vi "CRC-16.vi"(6 "Reflected":bool, 8 "FinalXorValue":u16 format="%04x", 9 "InitialCRC":u16 format="%04x", 10 "Polynomial":u16 format="%04x", 11 "DATA":u8[](array[numeric]) format="%02x") -> (3 "CRC":u16 format="%04x")   [LabVIEW 2021, in "LIN Frame Protection Addon Engine.lvlib"]
uses:
  LIN Frame Protection Addon Engine.lvlib
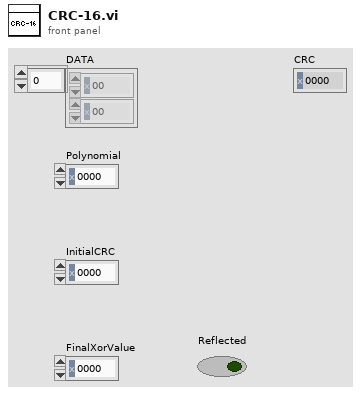
[diagram p1: front panel]
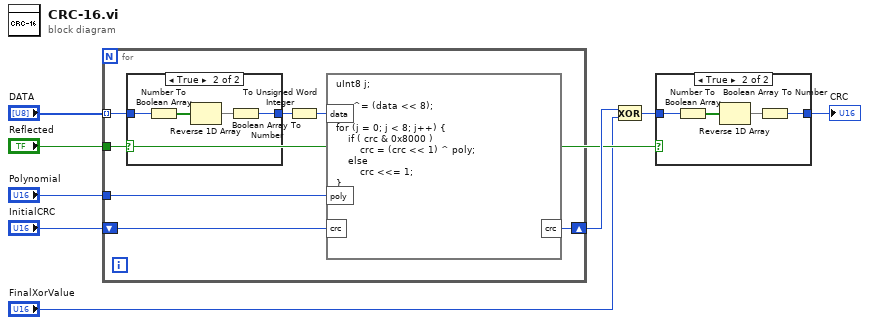
[diagram p0: block diagram]
diagram:
  n1 = for {
    tunnel: "Polynomial" -> [w15]
    tunnel: "DATA" -> [w11] mode=indexing
    tunnel: "Reflected" -> [w13]
    shift-right: [w10] -> w5
    shift-left: "InitialCRC" -> [w14]
    n2 = case shown="True" w13 {
      tunnel: [w16 w19] -> w12
      tunnel: w11 -> [w16 w20]
      frame False {
      }
      frame True {
        n3 = Number To Boolean Array(number=w20) -> (Boolean array=w18:bool[])
        n4 = Reverse 1D Array(array=w18) -> (reversed array=w17:bool[])
        n5 = Boolean Array To Number(Boolean array=w17) -> (number=w19:u8)
      }
    }
    n6 = To Unsigned Word Integer(number=w12) -> (unsigned 16bit integer=w9:u16)
    n7 = formula code="uInt8 j;\n\ncrc ^= (data << 8);\n\nfor (j = 0; j < 8; j++) {\n    if ( crc & 0x8000 )\n        crc = (crc << 1) ^ poly;\n    else\n        crc <<= 1;\n}"("poly"=w15, "data"=w9, "crc"=w14) -> ("crc"=w10:u16)
  }
  n8 = Exclusive Or(1:"FinalXorValue", 2:w5) -> (0:w2:u16)
  n9 = case shown="True" "Reflected" {
    tunnel: [w21 w24] -> w3
    tunnel: w2 -> [w21 w25]
    frame False {
    }
    frame True {
      n10 = Number To Boolean Array(number=w25) -> (Boolean array=w23:bool[])
      n11 = Reverse 1D Array(array=w23) -> (reversed array=w22:bool[])
      n12 = Boolean Array To Number(Boolean array=w22) -> (number=w24:u16)
    }
  }
  "CRC" <- w3
